vi "Insight_Send_Synch_Pulse.vi"(8 "error in (no error)":errorcluster, 11 "telnet connection":T1) -> (0 "error out":errorcluster, 1 "response data":string, 3 "telnet  connection out":T1)   [LabVIEW 2011]
doc: "Insight Photonic Solutions\n\nThis VI generates a short optical power pulse from the laser, for use in synchronizing the laser sweep with a data acquisition system.\n\nver 1.0 - original release\nver1.1 - Added output for response data buffer"
uses:
  Telnet Session.ctl
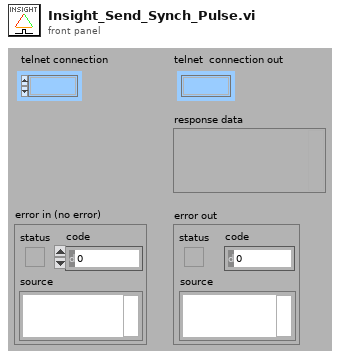
[diagram p1: front panel]
types:
  T1 = typedef "Telnet Session.ctl" = refnum<k1>
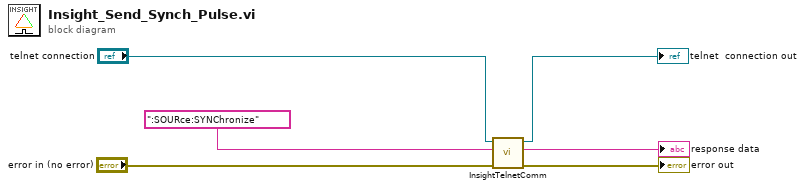
[diagram p0: block diagram]
diagram:
  n1 = call "InsightTelnetComm.vi"("error in"="error in (no error)", "write buffer (\"\")"=":SOURce:SYNChronize" ("String"), "telnet connection"="telnet connection") -> ("error out"=→"error out":errorcluster, "response data"=→"response data":string, "telnet  connection out"=→"telnet  connection out":T1)  [unwired: 4 in]
